vi "Anzeige Zustandsfelder.vi"() -> (0 "Zustand FID THC":u32, 1 "Zustand FID CH4":u32, 2 "Zustand NDIR lo":u32, 3 "Zustand FT-IR":u32, 4 "Zustand PMA":u32, 6 "BEENDEN":bool)   [LabVIEW 2020, in "Auto Kalibrieren.lvlib"]
uses:
  Auto Kalibrieren.lvlib
  Aktionen FGV Zustand Kalibrierung.ctl
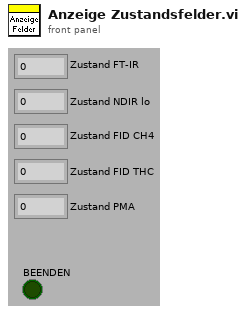
[diagram p1: front panel]
types:
  T1 = typedef "Auto Kalibrieren.lvlib/Aktionen FGV Zustand Kalibrierung.ctl" = enum16{"lesen", "LÖSCHEN", "Hintergrund fertig", "Nullpunkt NDIR CO lo", "Endpunkt NDIR CO lo", "Nullpunkt NDIR CO hi", "Endpunkt NDIR CO hi", "Nullpunkt NDIR CO2 lo", "Endpunkt NDIR CO2 lo", "Nullpunkt FID CH4", "Endpunkt FID CH4", "Nullpunkt FID THC", "Endpunkt FID THC", "Nullpunkt PMA", "Endpunkt PMA", "Fehler FT-IR", "Fehler NDIR lo", "Fehler FID CH4", "Fehler FID THC", "Fehler PMA", "TIMEOUT"}
  T2 = typedef "Auto Kalibrieren.lvlib/Zustand Messgeraete Kalibrierung.ctl" = cluster{"Hintergrund FT-IR":bool, "Nullpunkt NDIR CO lo":bool, "Endpunkt NDIR CO lo":bool, "Nullpunkt NDIR CO hi":bool, "Endpunkt NDIR CO hi":bool, "Nullpunkt NDIR CO2 lo":bool, "Endpunkt NDIR CO2 lo":bool, "Nullpunkt FID CH4":bool, "Endpunkt FID CH4":bool, "Nullpunkt FID THC":bool, "Endpunkt FID THC":bool, "Nullpunkt PMA":bool, "Endpunkt PMA":bool, "Fehler FT-IR":bool, "Fehler NDIR lo":bool, "Fehler FID CH4":bool, "Fehler FID THC":bool, "Fehler PMA":bool}
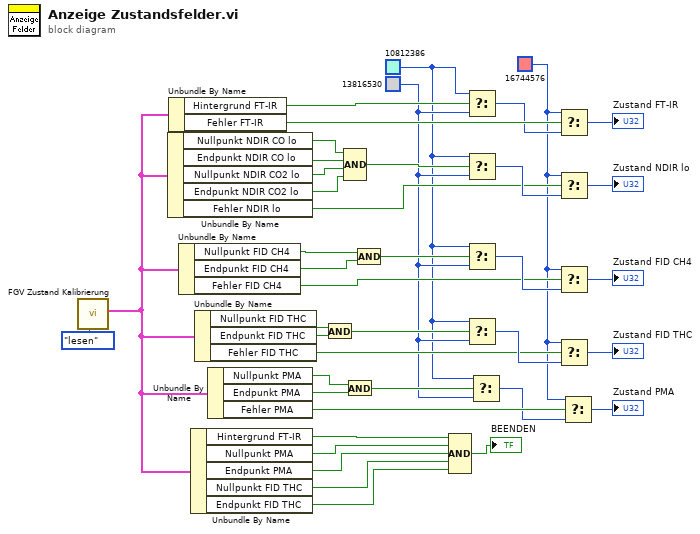
[diagram p0: block diagram]
diagram:
  w4 = u32 16744576 ("Farbfeld")
  w6 = u32 13816530 ("Farbfeld")
  w5 = u32 10812386 ("Farbfeld")
  n1 = call "FGV Zustand Kalibrierung.vi"("Aktionen"=Aktionen_FGV_Zustand_Kalibrierung."lesen" ("Enum")) -> ("Zustand Kalibrierung"=w7:T2)  [unwired: 9 in, 1 out]
  n2 = Unbundle By Name(w7) -> ("Nullpunkt NDIR CO lo"=w18:bool, "Endpunkt NDIR CO lo"=w19:bool, "Nullpunkt NDIR CO2 lo"=w39:bool, "Endpunkt NDIR CO2 lo"=w38:bool, "Fehler NDIR lo"=w26:bool)
  n3 = Unbundle By Name(w7) -> ("Hintergrund FT-IR"=w35:bool, "Fehler FT-IR"=w34:bool)
  n4 = Unbundle By Name(w7) -> ("Nullpunkt FID CH4"=w40:bool, "Endpunkt FID CH4"=w16:bool, "Fehler FID CH4"=w17:bool)
  n5 = Unbundle By Name(w7) -> ("Hintergrund FT-IR"=w15:bool, "Nullpunkt PMA"=w14:bool, "Endpunkt PMA"=w13:bool, "Nullpunkt FID THC"=w2:bool, "Endpunkt FID THC"=w1:bool)
  n6 = Unbundle By Name(w7) -> ("Nullpunkt FID THC"=w37:bool, "Endpunkt FID THC"=w36:bool, "Fehler FID THC"=w25:bool)
  n7 = Unbundle By Name(w7) -> ("Nullpunkt PMA"=w8:bool, "Endpunkt PMA"=w9:bool, "Fehler PMA"=w12:bool)
  n8 = And(x=w37, y=w36) -> (x .and. y?=w27:bool)
  n9 = Compound Arithmetic op=AND(w18, w19, w39, w38) -> (w28:bool)
  n10 = And(x=w8, y=w9) -> (x .and. y?=w11:bool)
  n11 = Compound Arithmetic op=AND(w40, w16) -> (w29:bool)
  n12 = Compound Arithmetic op=AND(w15, w14, w13, w2, w1) -> (→"BEENDEN":bool)
  n13 = Select(t=w5, s=w35, f=w6) -> (s? t:f=w33:u32)
  n14 = Select(t=w5, s=w28, f=w6) -> (s? t:f=w32:u32)
  n15 = Select(t=w5, s=w29, f=w6) -> (s? t:f=w31:u32)
  n16 = Select(t=w5, s=w27, f=w6) -> (s? t:f=w30:u32)
  n17 = Select(t=w5, s=w11, f=w6) -> (s? t:f=w10:u32)
  n18 = Select(t=w4, s=w34, f=w33) -> (s? t:f=→"Zustand FT-IR":u32)
  n19 = Select(t=w4, s=w26, f=w32) -> (s? t:f=→"Zustand NDIR lo":u32)
  n20 = Select(t=w4, s=w17, f=w31) -> (s? t:f=→"Zustand FID CH4":u32)
  n21 = Select(t=w4, s=w25, f=w30) -> (s? t:f=→"Zustand FID THC":u32)
  n22 = Select(t=w4, s=w12, f=w10) -> (s? t:f=→"Zustand PMA":u32)
